vi "packetizer.vi"(4 "invert":bool, 6 "data":u32[](array[numeric]) format="%x", 7 "countfields":u8=33, 8 "messagetype":u32=7168 format="%x", 9 "header":u32=43690 format="%x") -> (3 "output":string)   [LabVIEW 2014]
panel:
  in  "processingstring":string
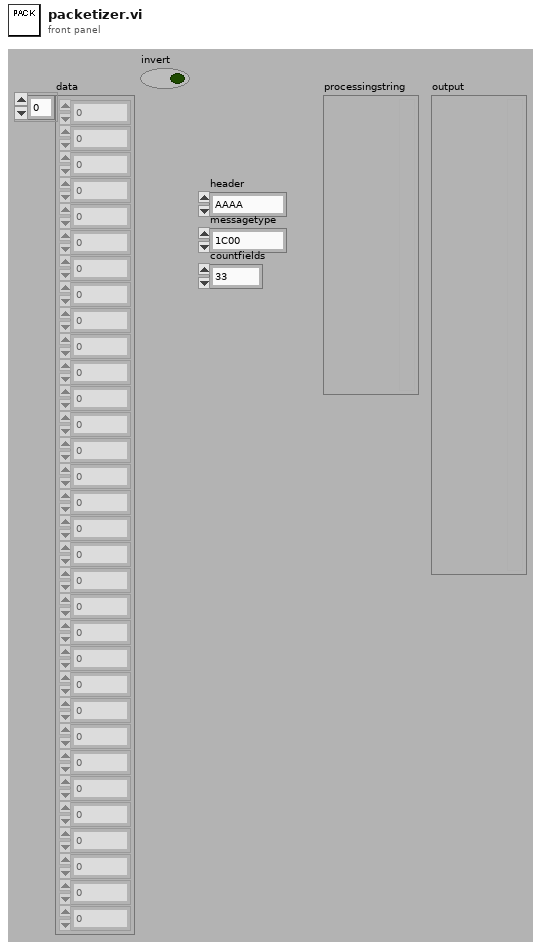
[diagram p1: front panel]
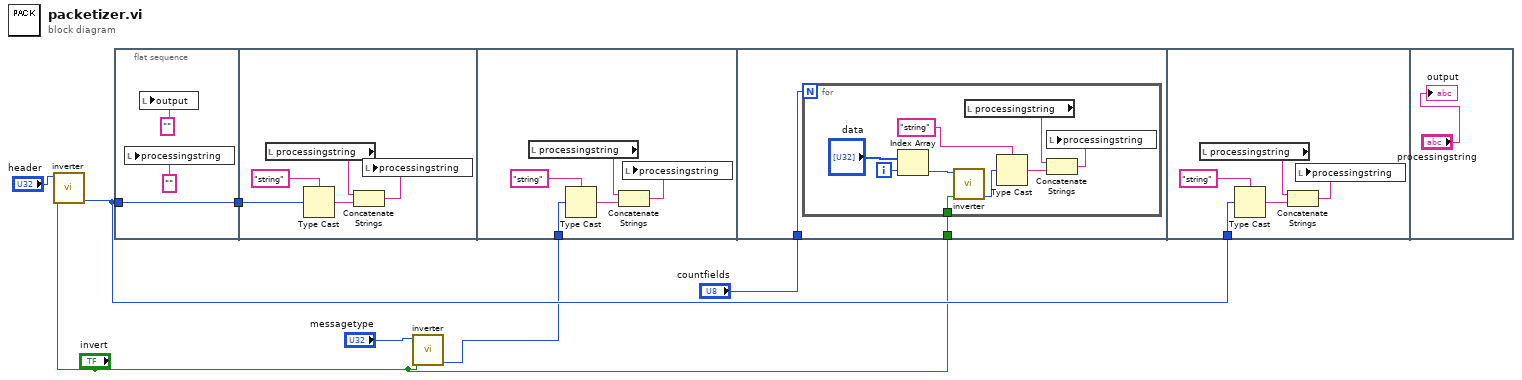
[diagram p0: block diagram]
diagram:
  n1 = call "inverter.vi"("invert"="invert", "input"="header") -> ("output"=w4:u32)  [unwired: 9 out]
  n2 = flat-sequence {
    tunnel: w4 -> [w10]
    tunnel: [w10] -> w6
    tunnel: w6 -> [w15]
    tunnel: w2 -> [w16]
    tunnel: "countfields" -> [w22]
    tunnel: "invert" -> [w21]
    tunnel: w4 -> [w32]
    frame #0 {
      n3 = local write "processingstring"("" ("output")) -> ()
      n4 = local write "output"("" ("output")) -> ()
    }
    frame #1 {
      n5 = local read "processingstring"() -> (w11:string)
      n6 = Type Cast(type="string", x=w15) -> (*(type *) &x=w12:string)
      n7 = Concatenate Strings(w11, w12) -> (w13:string)
      n8 = local write "processingstring"(w13) -> ()
    }
    frame #2 {
      n9 = local read "processingstring"() -> (w20:string)
      n10 = Type Cast(type="string", x=w16) -> (*(type *) &x=w19:string)
      n11 = Concatenate Strings(w20, w19) -> (w18:string)
      n12 = local write "processingstring"(w18) -> ()
    }
    frame #3 {
      n13 = for {
        N: w22 -> [_]
        tunnel: w21 -> [w25]
        i -> [w31]
        n14 = Index Array(array="data", index=w31) -> (element=w24:u32)
        n15 = call "inverter.vi"("invert"=w25, "input"=w24) -> ("output"=w23:u32)  [unwired: 9 out]
        n16 = local read "processingstring"() -> (w27:string)
        n17 = Type Cast(type="string", x=w23) -> (*(type *) &x=w28:string)
        n18 = Concatenate Strings(w27, w28) -> (w26:string)
        n19 = local write "processingstring"(w26) -> ()
      }
    }
    frame #4 {
      n20 = local read "processingstring"() -> (w36:string)
      n21 = Type Cast(type="string", x=w32) -> (*(type *) &x=w35:string)
      n22 = Concatenate Strings(w36, w35) -> (w34:string)
      n23 = local write "processingstring"(w34) -> ()
    }
    frame #5 {
      "output" <- "processingstring"
    }
  }
  n24 = call "inverter.vi"("invert"="invert", "input"="messagetype") -> ("output"=w2:u32)  [unwired: 9 out]
